vi "test Signed and Unsigned.vi"(8 "error in (no error)":errorcluster, 11 "TestCase in":refnum<class "BCD.lvclass">) -> (0 "error out":errorcluster, 3 "TestCase out":refnum<class "BCD.lvclass">)   [LabVIEW 2020, in "BCD.lvclass"]
uses:
  BCD.lvclass
  df3b5eb7-6bcb-40af-ab14-138a841d4224.vi
  e5a9ed8d-a936-4bcd-9e48-8176d125cb75.vi
  1fcb4e57-dc1d-4d3f-a87f-d06a729f5a18.vi
  5f41c702-736d-46cb-8ad7-d7a8da9834e5.vi
  df3b5eb7-6bcb-40af-ab14-138a841d4224.vi/a54b505c-1216-4ef4-8378-3ceda9d188df.vi
  df3b5eb7-6bcb-40af-ab14-138a841d4224.vi/136dcdcb-2dd3-4a4d-a796-a8f7a3f8e1ac.vi
  e5a9ed8d-a936-4bcd-9e48-8176d125cb75.vi/0a001d06-2809-4638-8d0b-e017d2157007.vi
  BCD Decode Integer.vi
  1fcb4e57-dc1d-4d3f-a87f-d06a729f5a18.vi/a54b505c-1216-4ef4-8378-3ceda9d188df.vi
  1fcb4e57-dc1d-4d3f-a87f-d06a729f5a18.vi/136dcdcb-2dd3-4a4d-a796-a8f7a3f8e1ac.vi
  5f41c702-736d-46cb-8ad7-d7a8da9834e5.vi/a54b505c-1216-4ef4-8378-3ceda9d188df.vi
  5f41c702-736d-46cb-8ad7-d7a8da9834e5.vi/136dcdcb-2dd3-4a4d-a796-a8f7a3f8e1ac.vi
  df3b5eb7-6bcb-40af-ab14-138a841d4224.vi/a54b505c-1216-4ef4-8378-3ceda9d188df.vi/a7fcce85-1f75-4572-aeaa-ddfd463a7c5f.vi
  BCD Decode Integer.vi/9a65bfc0-0d77-4ef3-ab58-63df1e1caa90.vi
  1fcb4e57-dc1d-4d3f-a87f-d06a729f5a18.vi/a54b505c-1216-4ef4-8378-3ceda9d188df.vi/a7fcce85-1f75-4572-aeaa-ddfd463a7c5f.vi
  5f41c702-736d-46cb-8ad7-d7a8da9834e5.vi/a54b505c-1216-4ef4-8378-3ceda9d188df.vi/a7fcce85-1f75-4572-aeaa-ddfd463a7c5f.vi
  <vilib>/addons/_JKI Toolkits/VI Tester/TestCase.llb/TestCase.lvclass
  C:/Program Files (x86)/National Instruments/LabVIEW 2020/vi.lib/addons/_JKI Toolkits/VI Tester/TestCase.llb/TestCase.lvclass
panel:
  out "BCD encoded value":bool[](array[boolean])
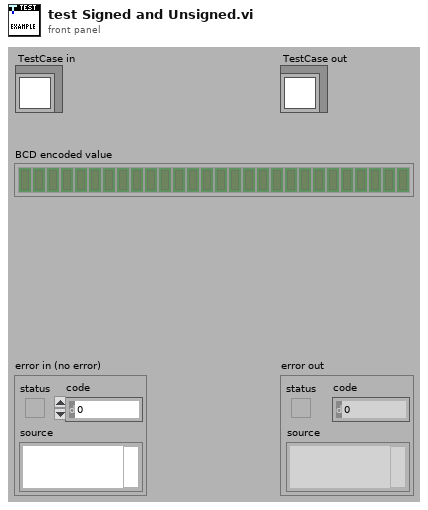
[diagram p1: front panel]
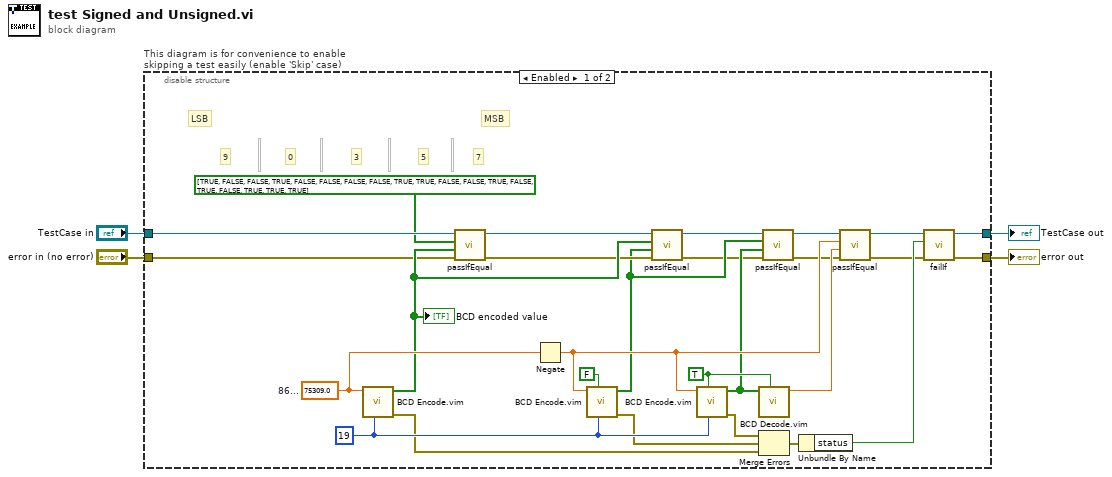
[diagram p0: block diagram]
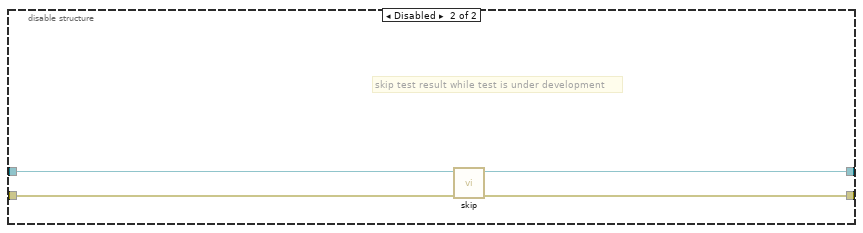
[diagram p2: hidden frame]
diagram:
  n1 = disable-structure "This diagram is for convenience to enable skipping a test easily (enable 'Skip' case)" shown="Enabled" {
    disable-tunnel: "TestCase in" -> [w24 w35]
    disable-tunnel: [w5 w33] -> w1
    disable-tunnel: [w6 w34] -> w3
    disable-tunnel: "error in (no error)" -> [w21 w32]
    frame Enabled {
      w28 = TRUE ("signed")
      w29 = 19 ("data size (bits)")
      w31 = 75309.0  # 86...
      # "MSB"
      # "LSB"
      # "9"
      # "0"
      # "3"
      # "5"
      # "7"
      n2 = call "BCD Encode.vim"("data size (bits)"=w29, "value"=w31) -> ("error out"=w11:errorcluster, "BCD encoded value"=w23:bool[])  [unwired: 7 in, 1 out]
      "BCD encoded value" <- w23
      n3 = call-dynamic "passIfEqual.vi"("error in (no error)"=w21, "y"=w23, "x"=bool[] [TRUE, FALSE, FALSE, TRUE, FALSE, FALSE, FALSE, FALSE, TRUE, TRUE, FALSE, FALSE, TRUE, FALSE, TRUE, FALSE, TRUE, TRUE, TRUE] ("BCD encoded value"), "TestCase in"=w24) -> ("error out"=w22:errorcluster, "TestCase out"=w25:refnum<class "BCD.lvclass">)  [unwired: 6 in]
      n4 = Negate(x=w31) -> (-x=w26:dbl)
      n5 = call "BCD Encode.vim"("data size (bits)"=w29, "signed"=FALSE, "value"=w26) -> ("error out"=w12:errorcluster, "BCD encoded value"=w19:bool[])  [unwired: 6 in, 1 out]
      n6 = call-dynamic "passIfEqual.vi"("error in (no error)"=w22, "y"=w19, "x"=w23, "TestCase in"=w25) -> ("error out"=w18:errorcluster, "TestCase out"=w17:refnum<class "BCD.lvclass">)  [unwired: 6 in]
      n7 = call "BCD Encode.vim"("data size (bits)"=w29, "signed"=w28, "value"=w26) -> ("error out"=w13:errorcluster, "BCD encoded value"=w20:bool[])  [unwired: 6 in, 1 out]
      n8 = call "BCD Decode.vim"("signed"=w28, "BCD encoded value"=w20) -> ("value"=w27:dbl)  [unwired: 9 in]
      n9 = Merge Errors(w13, w12, w11) -> (w10:errorcluster)
      n10 = call-dynamic "passIfEqual.vi"("error in (no error)"=w18, "y"=w20, "x"=w19, "TestCase in"=w17) -> ("error out"=w15:errorcluster, "TestCase out"=w16:refnum<class "BCD.lvclass">)  [unwired: 6 in]
      n11 = Unbundle By Name(w10) -> ("status"=w9:bool)
      n12 = call-dynamic "passIfEqual.vi"("error in (no error)"=w15, "y"=w27, "x"=w26, "TestCase in"=w16) -> ("error out"=w7:errorcluster, "TestCase out"=w8:refnum<class "BCD.lvclass">)  [unwired: 6 in]
      n13 = call-dynamic "failIf.vi"("error in (no error)"=w7, "fail"=w9, "TestCase in"=w8) -> ("error out"=w6:errorcluster, "TestCase out"=w5:refnum<class "BCD.lvclass">)  [unwired: 7 in]
    }
    frame Disabled {
      # "skip test result while test is under development"
      n14 = call <vilib>:"skip.vi"("error in (no error)"=w32, "TestCase in"=w35) -> ("error out"=w34:errorcluster, "TestCase out"=w33:refnum<class "BCD.lvclass">)  [unwired: 8 in]
    }
  }
  "error out" <- w3
  "TestCase out" <- w1
